vi "Sample Push go for Stash State.vi"(8 "error in (no error)":errorcluster, 11 "cRIO-CO2 in":refnum<class "cRIO-CO2.lvclass">) -> (0 "error out":errorcluster, 3 "cRIO-CO2 out":refnum<class "cRIO-CO2.lvclass">)   [LabVIEW 2015, in "cRIO-Carbondioxide.lvlib" / "cRIO-CO2.lvlib" / "cRIO-CO2.lvclass"]
uses:
  cRIO-CO2.lvclass
  cRIO-CO2.lvclass/cRIO-CO2.ctl
  Controls/Sample Push State Enumerator.ctl
  State Elapsed Time.vi
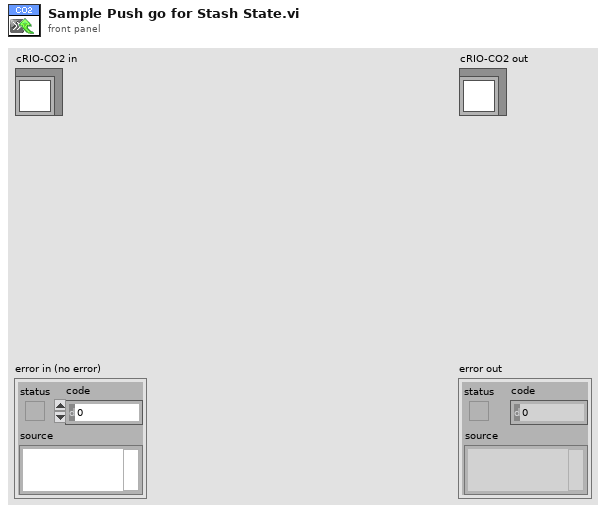
[diagram p1: front panel]
types:
  T1 = typedef "Sample Push State Enumerator.ctl" = enum16{"Undefined", "Initialize", "Dilute", "Close Transfer Line", "Start Heaters", "Warm Up Syringe", "Ready to Push", "Push", "Initiate Stash", "Stash", "Complete", "Abort", "Idle", "Error"}
  T2 = typedef "Sample Transfer State Enumerator.ctl" = enum16{"Idle", "Initialize", "Check Containers", "Check Temperatures", "Start Turbo", "Warm Up Containers", "Prepare for purging", "Purge Capillary", "Purge", "Open Containers", "Introduce Sample", "Measure Base Pressure", "Home Syringe", "Start Freezer", "Freeze Target", "Crystalize", "Initiate Stash", "Stash", "Polish", "Stop Freezers", "Push Sample", "Complete", "Abort", "Error", "Undefined"}
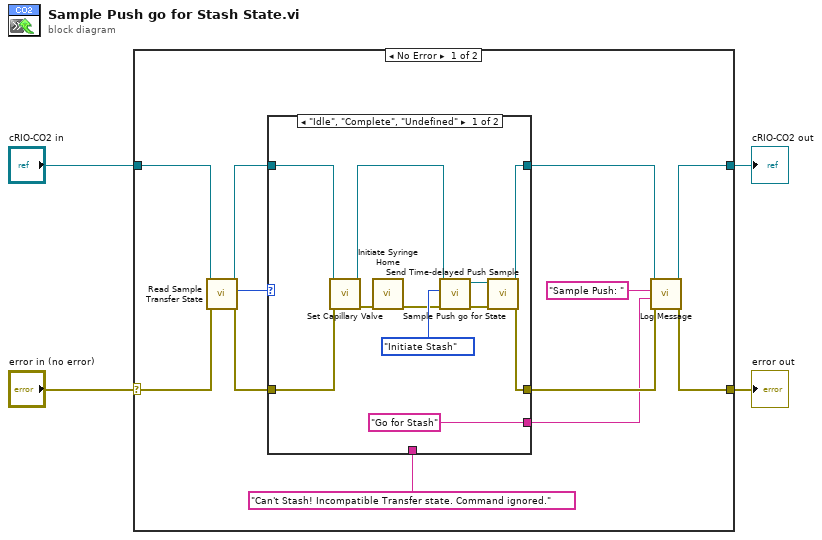
[diagram p0: block diagram]
diagram:
  n1 = case shown="No Error" "error in (no error)" {
    selector: "error in (no error)" -> [w16 w32]
    tunnel: [w10 w32] -> w3
    tunnel: [w8 w31] -> w1
    tunnel: "cRIO-CO2 in" -> [w15 w31]
    frame No Error {
      n2 = call "Read Sample Transfer State.vi"("error in (no error)"=w16, "cRIO-CO2 in"=w15) -> ("error out"=w5:errorcluster, "Sample Transfer State"=w13:T2, "cRIO-CO2 out"=w14:refnum<class "cRIO-CO2.lvclass">)  [unwired: 4 in, 3 out]
      n3 = case shown="\"Idle\", \"Complete\", \"Undefined\"" w13 {
        tunnel: w5 -> [w20 w29]
        tunnel: [w23 w29] -> w11
        tunnel: w14 -> [w18 w30]
        tunnel: [w21 w30] -> w9
        tunnel: ["Go for Stash" ("String") w28] -> w7
        tunnel: "Can't Stash! Incompatible Transfer state. Command ignored." ("String") -> [_ w28]
        frame "Idle", "Complete", "Undefined" {
          n4 = call "Set Capillary Valve.vi"("error in (no error)"=w20, "cRIO-CO2 in"=w18) -> ("error out"=w19:errorcluster, "cRIO-CO2 out"=w17:refnum<class "cRIO-CO2.lvclass">)  [unwired: 8 in]
          n5 = call "Initiate Syringe Home.vi"("error in (no error)"=w19) -> ("error out"=w25:errorcluster)  [unwired: 10 in]
          n6 = call "Sample Push go for State.vi"("error in (no error)"=w25, "Sample Push State"=Sample_Push_State_Enumerator."Initiate Stash", "cRIO-CO2 in"=w17) -> ("error out"=w24:errorcluster, "cRIO-CO2 out"=w22:refnum<class "cRIO-CO2.lvclass">)  [unwired: 7 in]
          n7 = call "Send Time-delayed Push Sample.vi"("error in (no error)"=w24, "cRIO-CO2 in"=w22) -> ("error out"=w23:errorcluster, "cRIO-CO2 out"=w21:refnum<class "cRIO-CO2.lvclass">)  [unwired: 8 in]
        }
        frame "Purge Capillary", Default {
        }
      }
      n8 = call "Log Message.vi"("error in (no error)"=w11, "String"=w7, "Source Name"="Sample Push: ", "cRIO-CO2 in"=w9) -> ("error out"=w10:errorcluster, "cRIO-CO2 out"=w8:refnum<class "cRIO-CO2.lvclass">)  [unwired: 6 in]
    }
    frame Error {
    }
  }
  "error out" <- w3
  "cRIO-CO2 out" <- w1
